vi "Read_TestItem.vi"(8 "error in (no error)":errorcluster caption="错误输入（无错误）", 10 "组合框":string(combo), 11 "path":path caption="路径") -> (0 "error out":errorcluster, 2 "OutData":string[](array[string]), 3 "path 2":path caption="路径")   [LabVIEW 2018]
uses:
  <vilib>/Utility/config.llb/Read Key (String).vi
  <vilib>/Utility/config.llb/NI_LVConfig.lvlib
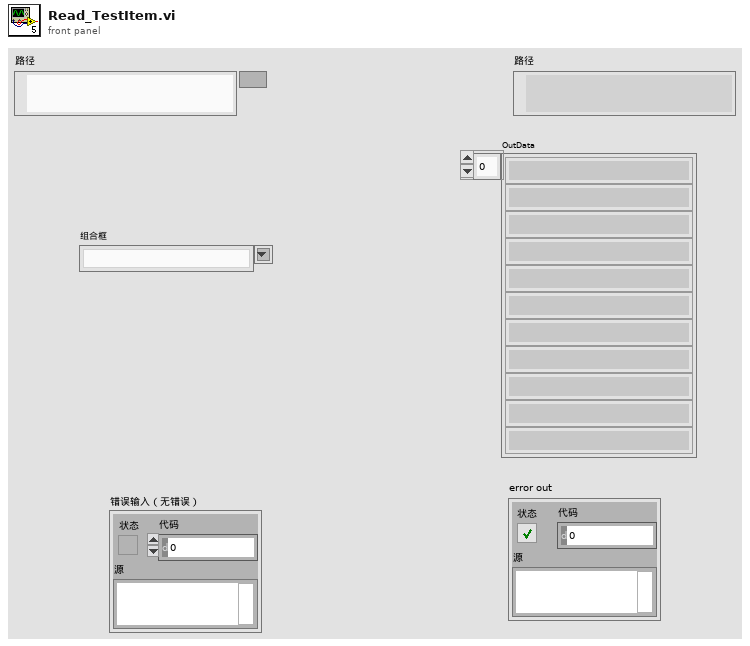
[diagram p1: front panel]
types:
  T1 = typedef "NI_LVConfig.lvlib/Config Data RefNum.ctl" = refnum<k1>
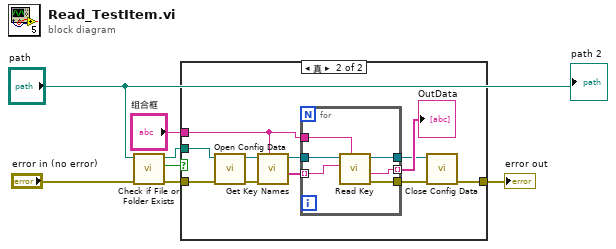
[diagram p0: block diagram]
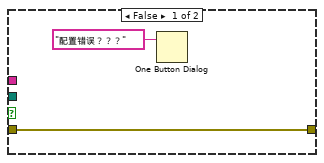
[diagram p2: hidden frame]
diagram:
  n1 = call <vilib>:"Check if File or Folder Exists.vi"("error in (no error)"="error in (no error)", "path"="path") -> ("error out"=w4:errorcluster, "file or folder exists?"=w2:bool, "dup path"=w3:path)  [unwired: 7 in]
  n2 = case shown="真" w2 {
    tunnel: w3 -> [_ w20]
    tunnel: w4 -> [w8 w19]
    tunnel: "组合框" -> [_ w13]
    tunnel: [w8 w10] -> w6
    frame False {
      n3 = One Button Dialog(message="配置错误？？？" ("消息")) -> ()  [unwired: 1 in, 1 out]
    }
    frame True {
      n4 = call <vilib>:"Open Config Data.vi"("error in (no error)"=w19, "configuration file path"=w20) -> ("error out"=w17:errorcluster, "refnum"=w18:T1)  [unwired: 7 in, 1 out]
      n5 = call <vilib>:"Get Key Names.vi"("section"=w13, "error in (no error)"=w17, "refnum"=w18) -> ("key names"=w15:string[], "refnum out"=w16:T1)  [unwired: 5 in, 2 out]
      n6 = for {
        tunnel: w16 -> [w26]
        tunnel: w15 -> [w25] mode=indexing
        tunnel: [w24] -> w14 mode=indexing
        tunnel: w13 -> [w23]
        tunnel: [w22] -> w12
        tunnel: [w21] -> w11
        n7 = call-poly <vilib>:"Read Key.vi"("section"=w23, "key"=w25, "refnum"=w26) -> ("error out"=w21:errorcluster, "value"=w24:string, "refnum out"=w22:T1)  [unwired: 5 in, 1 out]
      }
      "OutData" <- w14
      n8 = call <vilib>:"Close Config Data.vi"("error in (no error)"=w11, "refnum"=w12) -> ("error out"=w10:errorcluster)  [unwired: 8 in, 1 out]
    }
  }
  "error out" <- w6
  "path 2" <- "path"
